vi "SDCP SMF Rx Logger - Notifier FGV.vi"(4 "error in (no error)":errorcluster, 5 "Command":T2, 6 "Notifier name":T1, 7 "Notifier value in":variant) -> (0 "error out":errorcluster, 3 "Notifier value out":variant)   [LabVIEW 2020]
uses:
  Typedefs/SDCP SMF Rx Logger - Notifier FGV - Commands.ctl
  Typedefs/SDCP SMF Rx Logger - Notifier FGV - Notifier names.ctl
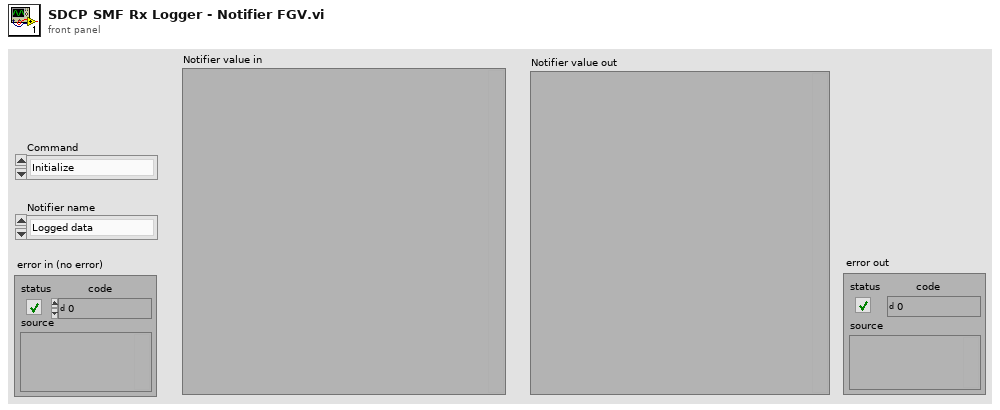
[diagram p1: front panel]
types:
  T1 = typedef "SDCP SMF Rx Logger - Notifier FGV - Notifier names.ctl" = enum16{"Logged data", "Pause logging", "Get log", "Reset log", "Sample counter", "Logged data buffer", "Stop logging"}
  T2 = typedef "SDCP SMF Rx Logger - Notifier FGV - Commands.ctl" = enum16{"Initialize", "Read", "Write", "Deinitialize"}
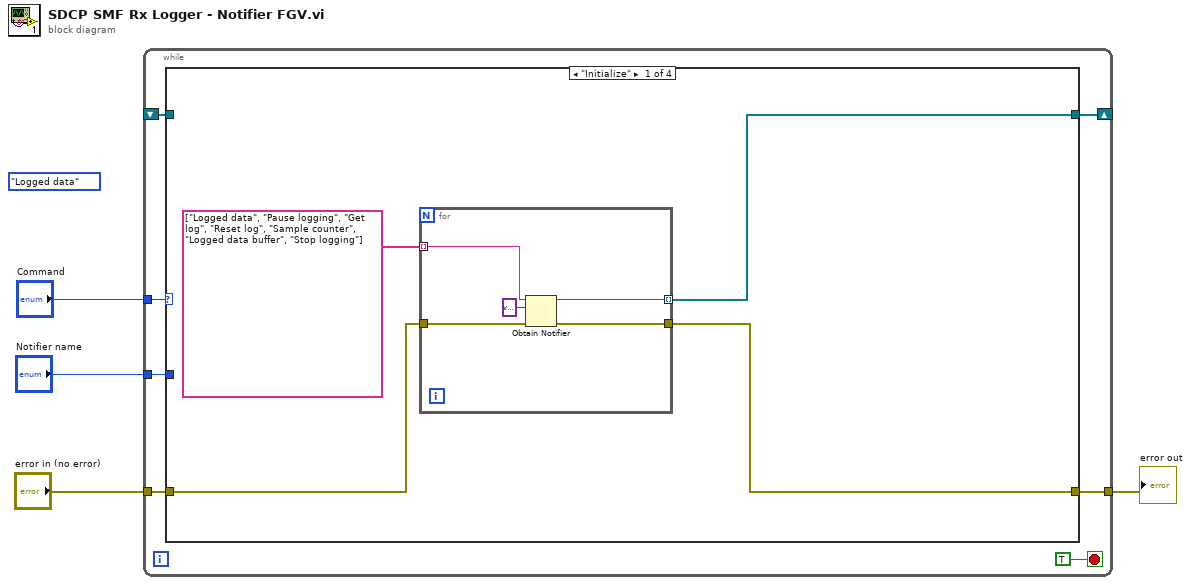
[diagram p0: block diagram]
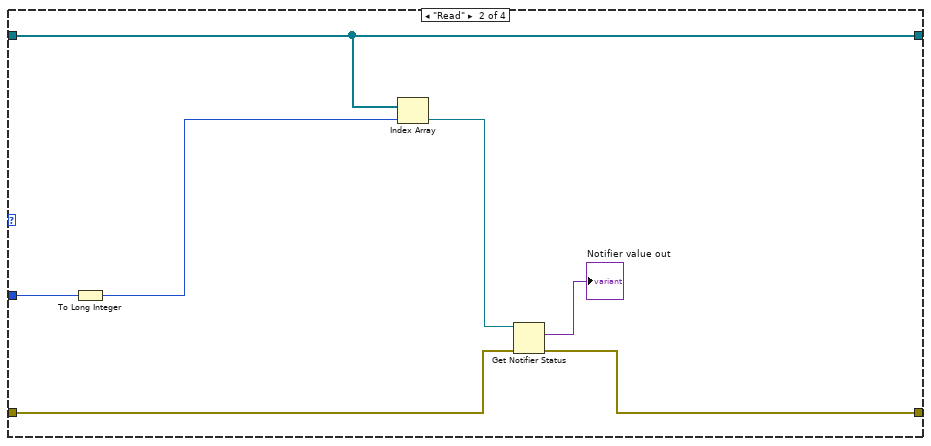
[diagram p2: hidden frame]
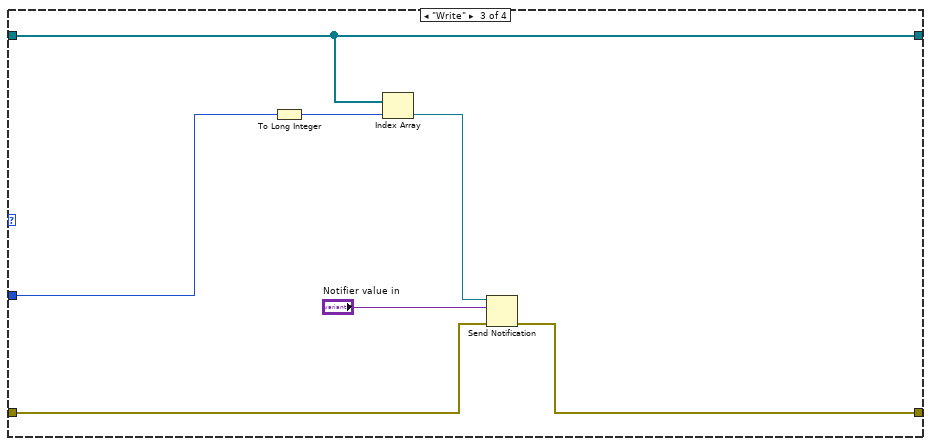
[diagram p3: hidden frame]
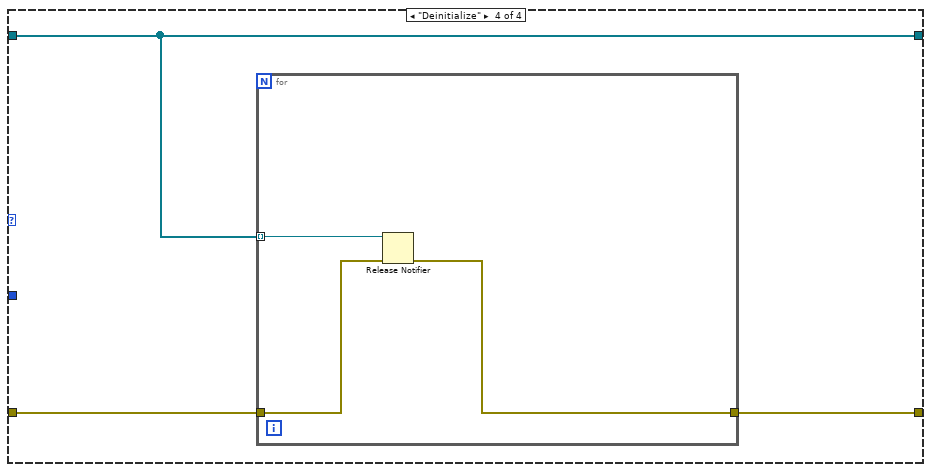
[diagram p4: hidden frame]
diagram:
  (unwired) SDCP_SMF_Rx_Logger_-_Notifier_FGV_-_Notifier_names."Logged data" ("Notifier name")
  n1 = while {
    tunnel: "error in (no error)" -> [w9]
    tunnel: "Command" -> [w11]
    tunnel: [w8] -> w2
    shift-right: [w7] -> _
    shift-left: _ -> [w6]
    tunnel: "Notifier name" -> [w5]
    stop <- TRUE stop-if-true
    n2 = case shown="\"Initialize\"" w11 {
      tunnel: w9 -> [w15 w23 w30 w37]
      tunnel: [w14 w22 w29 w36] -> w8
      tunnel: [w12 w27 w34 w35] -> w7
      tunnel: w6 -> [_ w27 w34 w35]
      tunnel: w5 -> [_ w26 w33 _]
      frame "Initialize" {
        n3 = for {
          tunnel: w15 -> [w20]
          tunnel: [w19] -> w14
          tunnel: string[] ["Logged data", "Pause logging", "Get log", "Reset log", "Sample counter", "Logged data buffer", "Stop logging"] -> [w17] mode=indexing
          tunnel: [w16] -> w12 mode=indexing
          n4 = Obtain Notifier(name (unnamed)=w17, notification data type=variant ("element data type"), error in (no error)=w20) -> (notifier out=w16:refnum<notifier>, error out=w19:errorcluster)  [unwired: 1 in, 1 out]
        }
      }
      frame "Read" {
        n5 = To Long Integer(number=w26) -> (32bit integer=w25:i32)
        n6 = Index Array(array=w27, index=w25) -> (element=w24:refnum<notifier>)
        n7 = Get Notifier Status(notifier=w24, error in (no error)=w23) -> (current notification=→"Notifier value out":variant, error out=w22:errorcluster)  [unwired: 3 out]
      }
      frame "Write" {
        n8 = To Long Integer(number=w33) -> (32bit integer=w32:i32)
        n9 = Index Array(array=w34, index=w32) -> (element=w31:refnum<notifier>)
        n10 = Send Notification(notification="Notifier value in", notifier=w31, error in (no error)=w30) -> (error out=w29:errorcluster)  [unwired: 1 out]
      }
      frame "Deinitialize" {
        n11 = for {
          tunnel: w37 -> [w39]
          tunnel: [w38] -> w36
          tunnel: w35 -> [w40] mode=indexing
          n12 = Release Notifier(notifier=w40, error in (no error)=w39) -> (error out=w38:errorcluster)  [unwired: 1 in, 2 out]
        }
      }
    }
  }
  "error out" <- w2
